vi "makeClampWvfrm_VcmdtoV.vi"(11 "voltage in (mV)":dbl) -> (3 "cmd voltage (V)":dbl)   [LabVIEW 2019]
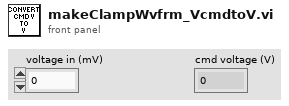
[diagram p1: front panel]
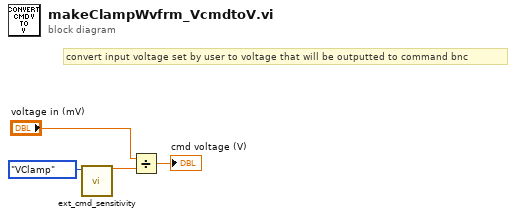
[diagram p0: block diagram]
diagram:
  # "convert input voltage set by user to voltage that will be outputted to command bnc"
  n1 = call "ext_cmd_sensitivity.vi"("which clamp"=enum16{"VClamp", "IClamp"}."VClamp") -> ("division factor"=w1:dbl)  [unwired: 10 in]
  n2 = Divide(x="voltage in (mV)", y=w1) -> (x/y=→"cmd voltage (V)":dbl)
